vi "Trim Whitespace - Remove Space Before or After a String.vi"() -> ()   [LabVIEW 2016]
uses:
  <vilib>/Utility/error.llb/whitespace.ctl
panel:
  out "String 2":string
  in  "String":string
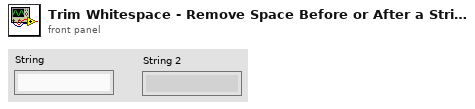
[diagram p1: front panel]
types:
  T1 = typedef "whitespace.ctl" = u16
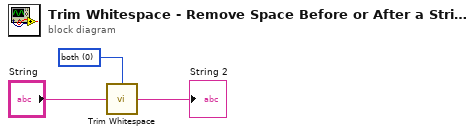
[diagram p0: block diagram]
diagram:
  w1 = T1 0 items=["both", "start of string", "end of string"] ("location (both)")
  n1 = call <vilib>:"Trim Whitespace.vi"("string"="String", "location (both)"=w1) -> ("trimmed string"=→"String 2":string)
